vi "RTS Macro Filter Compressor Peaks.vi"(0 "Refrigeration Full Data":T1, 11 "Error In":errorcluster) -> (4 "Refrigeration Full Data Output":T1, 6 "Refrigeration Core Stats":T2 {"Average Compressor Cycle Time (Min)" format="%0.2f"; "Average Compressor Power (W)" format="%0.2f"; "Power Start Time (sec)" format="%<%H:%M:%S>t"; "Power End time (sec)" format="%<%H:%M:%S>t"; "Average Defrost Power (W)" format="%0.2f"}, 13 "Transistion Index Locations":i32[](array[numeric]), 14 "Average Compressor Power (Lower)":dbl, 15 "Error Out":errorcluster)   [LabVIEW 2016]
uses:
  Type Definitions/RTS Macro Refrigeration Core Stats.ctl
  Type Definitions/RTS Macro Full Data.ctl
panel:
  out "Time @ Index":dbl[](array[numeric]) format="%<%H:%M:%S>t"
  out "Lower 3 Sig Limit":dbl
  out "Upper 3 Sig Limit":dbl
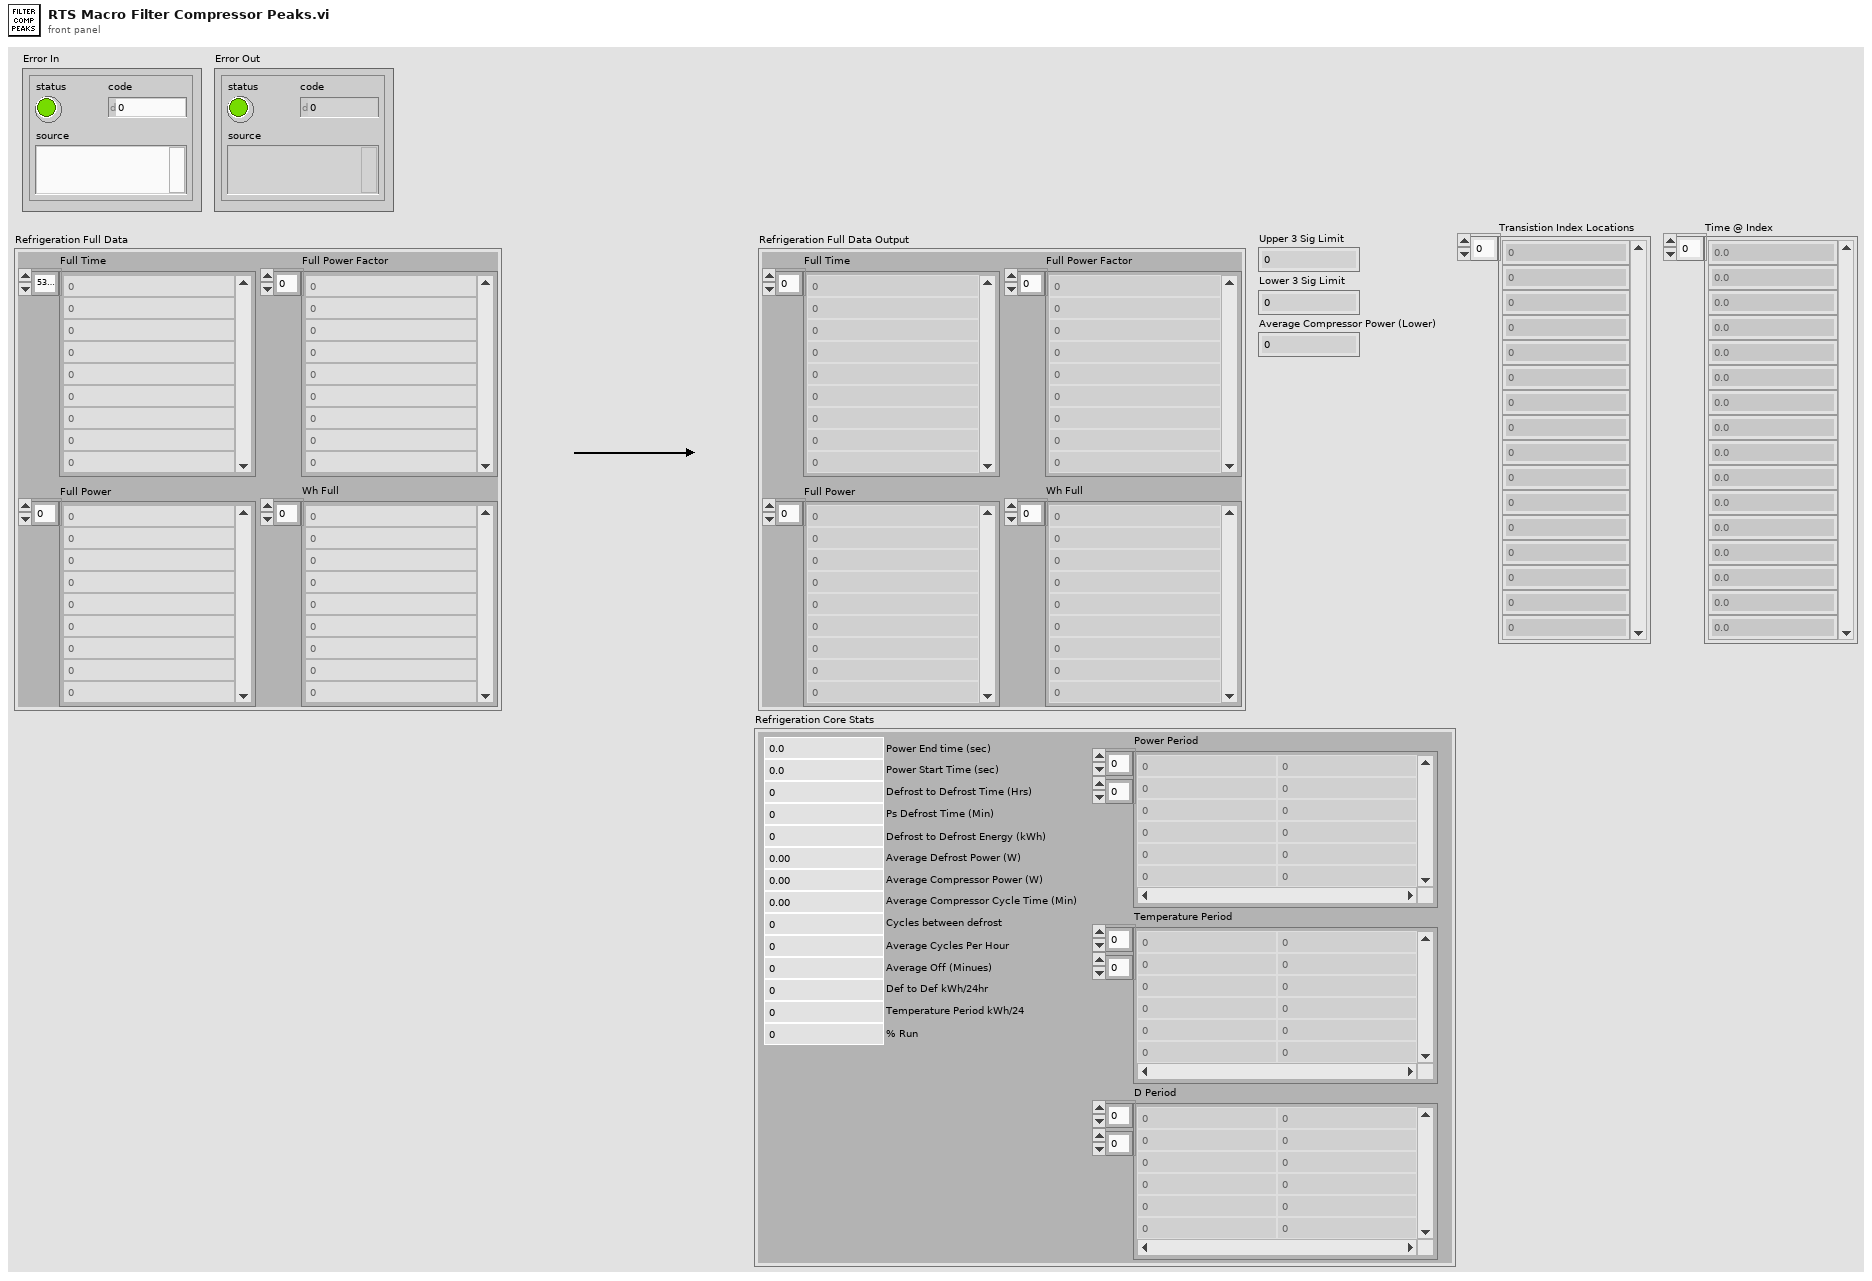
[diagram p1: front panel]
types:
  T1 = typedef "RTS Macro Full Data.ctl" = cluster{"Full Time":dbl[], "Full Power Factor":dbl[], "Full Power":dbl[], "Wh Full":dbl[]}
  T2 = typedef "RTS Macro Refrigeration Core Stats.ctl" = cluster{"Average Defrost Power (W)":dbl, "Power End time (sec)":dbl, "Power Start Time (sec)":dbl, "Defrost to Defrost Time (Hrs)":dbl, "Ps Defrost Time (Min)":dbl, "Defrost to Defrost Energy (kWh)":dbl, "Average Compressor Power (W)":dbl, "Average Compressor Cycle Time (Min)":dbl, "Power Period":dbl[][], "Cycles between defrost":i32, "Average Cycles Per Hour":dbl, "Average Off (Minues)":dbl, "Def to Def kWh/24hr":dbl, "Temperature Period kWh/24":dbl, "% Run":dbl, "Temperature Period":dbl[][], "D Period":dbl[][]}
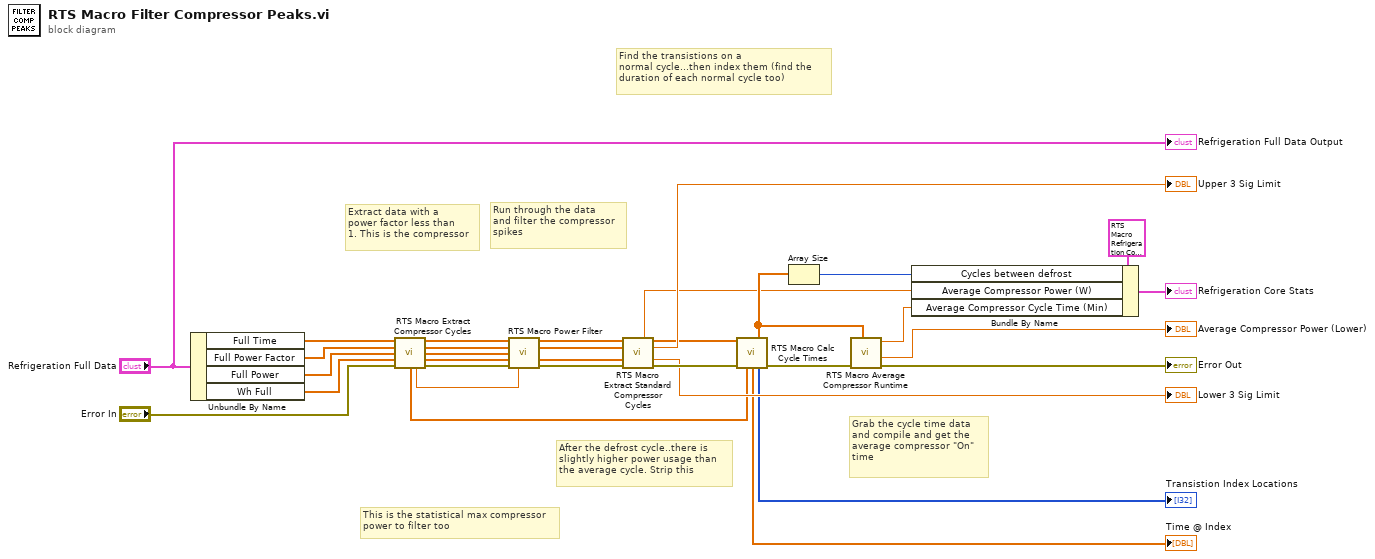
[diagram p0: block diagram]
diagram:
  # "Extract data with a \npower factor less than\n1. This is the compressor"
  # "This is the statistical max compressor\npower to filter too"
  # "Grab the cycle time data\nand compile and get the \naverage compressor \"On\"\ntime"
  # "Find the transistions on a \nnormal cycle...then index them (find the\nduration of each normal cycle too)"
  # "After the defrost cycle..there is \nslightly higher power usage than\nthe average cycle. Strip this"
  # "Run through the data\nand filter the compressor\nspikes"
  n1 = Unbundle By Name("Refrigeration Full Data") -> ("Full Time"=w10:dbl[], "Full Power Factor"=w9:dbl[], "Full Power"=w8:dbl[], "Wh Full"=w7:dbl[])
  n2 = call "RTS Macro Extract Compressor Cycles.vi"("Full Time"=w10, "Full Power Factor Data"=w9, "Full Power Data"=w8, "Full WH Data"=w7, "Error In"="Error In") -> ("Filtered Time"=w16:dbl[], "Filtered Power Factor"=w15:dbl[], "Filtered Power Data"=w14:dbl[], "Filtered Wh Data"=w13:dbl[], "Filtered Pulse Train"=w2:dbl[], "Top Compressor Range Data"=w19:dbl, "Error Out"=w18:errorcluster)  [unwired: 4 in]
  n3 = call "RTS Macro Power Filter.vi"("Filtered Time"=w16, "Filtered Power Factor"=w15, "Filtered Power Data"=w14, "Filtered Wh Data"=w13, "Error In"=w18, "Top Compressor Range Data"=w19) -> ("Time Output"=w32:dbl[], "Power Output"=w31:dbl[], "Power Factor Output"=w30:dbl[], "Error Out"=w21:errorcluster)  [unwired: 6 in]
  n4 = call "RTS Macro Extract Standard Compressor Cycles.vi"("Time"=w32, "Power (W)"=w31, "Power Factor"=w30, "Error In"=w21) -> ("Average Compressor Power (Watts)"=w5:dbl, "Standard Compressor Cycles Times"=w27:dbl[], "Upper 3 Sig Limit"=→"Upper 3 Sig Limit":dbl, "Lower 3 Sig Limit"=→"Lower 3 Sig Limit":dbl, "Error Out"=w26:errorcluster)  [unwired: 7 in]
  n5 = call "RTS Macro Calc Cycle Times.vi"("Time"=w27, "Error In"=w26, "Filtered Pulse Train"=w2) -> ("Defrost/Cycle Times"=w12:dbl[], "Time @ Index"=→"Time @ Index":dbl[], "Transistion Index Locations"=→"Transistion Index Locations":i32[], "Error Out"=w22:errorcluster)  [unwired: 8 in, 1 out]
  n6 = Array Size(array=w12) -> (size(s)=w4:i32)
  n7 = call "RTS Macro Average Compressor Runtime.vi"("Defrost/Cycle Times"=w12, "Error In"=w22) -> ("Error Out"=→"Error Out":errorcluster, "Average Compressor Power (Lower)"=→"Average Compressor Power (Lower)":dbl, "Average Compressor Cycle Time (Min)"=w24:dbl)  [unwired: 6 in, 1 out]
  n8 = Bundle By Name(cluster=T2 {"Average Defrost Power (W)"=0.0, "Power End time (sec)"=0.0, "Power Start Time (sec)"=0.0, "Defrost to Defrost Time (Hrs)"=0.0, "Ps Defrost Time (Min)"=0.0, "Defrost to Defrost Energy (kWh)"=0.0, "Average Compressor Power (W)"=0.0, "Average Compressor Cycle Time (Min)"=0.0, "Power Period"=[], "Cycles between defrost"=0, "Average Cycles Per Hour"=0.0, "Average Off (Minues)"=0.0, "Def to Def kWh/24hr"=0.0, "Temperature Period kWh/24"=0.0, "% Run"=0.0, "Temperature Period"=[], "D Period"=[]} ("Refrigeration Core Stats"), "Cycles between defrost"=w4, "Average Compressor Power (W)"=w5, "Average Compressor Cycle Time (Min)"=w24) -> (→"Refrigeration Core Stats":T2)
  "Refrigeration Full Data Output" <- "Refrigeration Full Data"
